vi "WPI_PWMConvertDeadbandMillisecondTimeTo8Bit.vi"(0 "DIO Loop Timing (ticks)":u16=261, 7 "PWMDeadband (ms)":T2) -> (8 "PWMDeadband Coefficient":T1)   [LabVIEW 2017]
uses:
  <vilib>/Rock Robotics/WPI/PWM/WPI_PWMDeadband_ms.ctl
  <vilib>/Rock Robotics/WPI/PWM/WPI_PWMDeadband.ctl
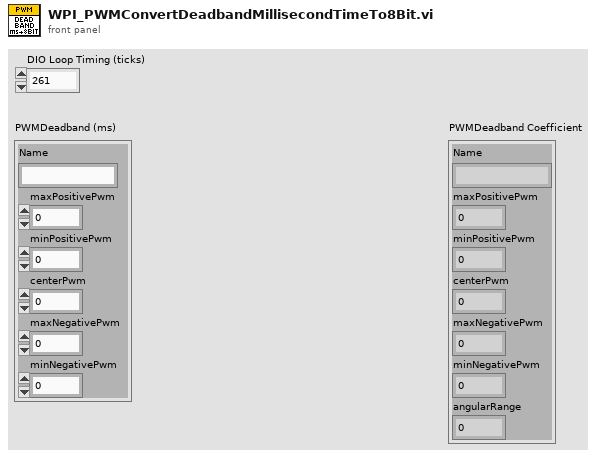
[diagram p1: front panel]
types:
  T1 = typedef "WPI_PWMDeadband.ctl" = cluster{"Name":string, "maxPositivePwm":i32, "minPositivePwm":i32, "centerPwm":i32, "maxNegativePwm":i32, "minNegativePwm":i32, "angularRange":u16}
  T2 = typedef "WPI_PWMDeadband_ms.ctl" = cluster{"Name":string, "maxPositivePwm":dbl, "minPositivePwm":dbl, "centerPwm":dbl, "maxNegativePwm":dbl, "minNegativePwm":dbl}
  T3 = cluster{"Name":string, "maxPositivePwm":i32, "minPositivePwm":i32, "centerPwm":i32, "maxNegativePwm":i32, "minNegativePwm":i32, "angularRange":u16}
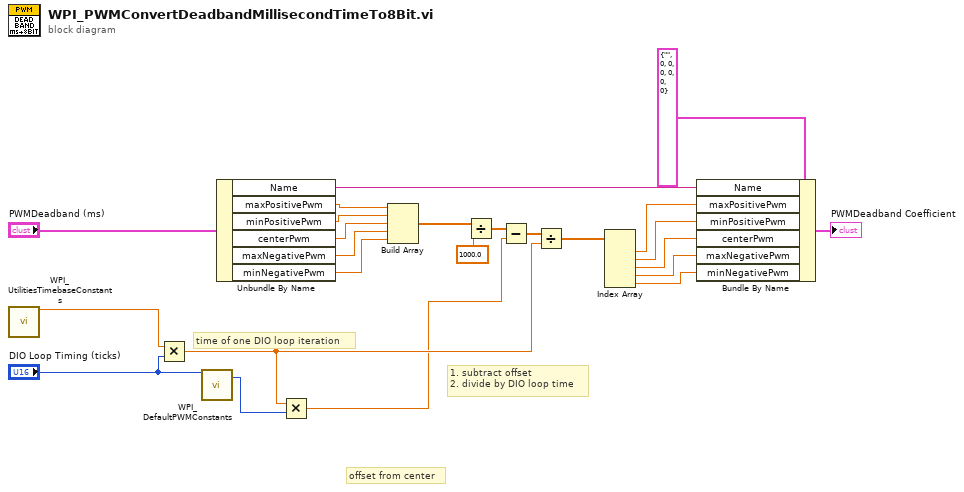
[diagram p0: block diagram]
diagram:
  # "offset from center"
  # "time of one DIO loop iteration"
  # "1. subtract offset\n2. divide by DIO loop time"
  n1 = call <vilib>:"WPI_UtilitiesTimebaseConstants.vi"() -> ("40 MHz FPGA clock"=w1:dbl)  [unwired: 13 in, 2 out]
  n2 = Multiply(x=w1, y="DIO Loop Timing (ticks)") -> (x*y=w17:dbl)
  n3 = call <vilib>:"WPI_DefaultPWMConstants.vi"("DIO Loop Timing (ticks)"="DIO Loop Timing (ticks)") -> ("defaultMinPWMHigh"=w2:u16)  [unwired: 16 in, 2 out]
  n4 = Unbundle By Name("PWMDeadband (ms)") -> ("Name"=w15:string, "maxPositivePwm"=w23:dbl, "minPositivePwm"=w22:dbl, "centerPwm"=w21:dbl, "maxNegativePwm"=w20:dbl, "minNegativePwm"=w19:dbl)
  n5 = Multiply(x=w17, y=w2) -> (x*y=w4:dbl)
  n6 = Build Array(w23, w22, w21, w20, w19) -> (w18:dbl[])
  n7 = Divide(x=w18, y=1000.0) -> (x/y=w6:dbl[])
  n8 = Subtract(x=w6, y=w4) -> (x-y=w7:dbl[])
  n9 = Divide(x=w7, y=w17) -> (x/y=w13:dbl[])
  n10 = Index Array(array=w13) -> (element #1=w12:dbl, element #2=w11:dbl, element #3=w10:dbl, element #4=w9:dbl, element #5=w8:dbl)  [unwired: 5 in]
  n11 = Bundle By Name(cluster=T3 {"Name"="", "maxPositivePwm"=0, "minPositivePwm"=0, "centerPwm"=0, "maxNegativePwm"=0, "minNegativePwm"=0, "angularRange"=0} ("PWMDeadband Coefficient"), "Name"=w15, "maxPositivePwm"=w12, "minPositivePwm"=w11, "centerPwm"=w10, "maxNegativePwm"=w9, "minNegativePwm"=w8) -> (→"PWMDeadband Coefficient":T3)
